vi "Open_File_Simple.vi"(6 "Read Only?":bool, 8 "error in (no error)":errorcluster, 9 "Overwrite?":bool, 10 "Path relative?":bool, 11 "Path":string) -> (0 "error out":errorcluster, 3 "refnum out":refnum<file>)   [LabVIEW 2016]
uses:
  <vilib>/Utility/error.llb/Error Cluster From Error Code.vi
  <vilib>/ErrorRing/Error Ring.xnode
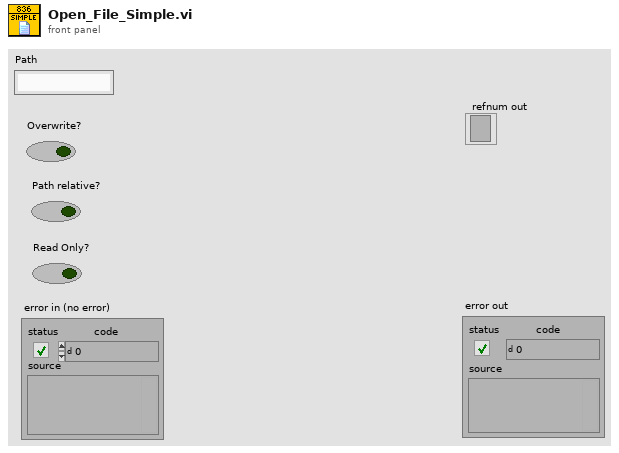
[diagram p1: front panel]
types:
  T1 = enum16{"open", "replace", "create", "open or create", "replace or create", "replace or create with confirmation"}
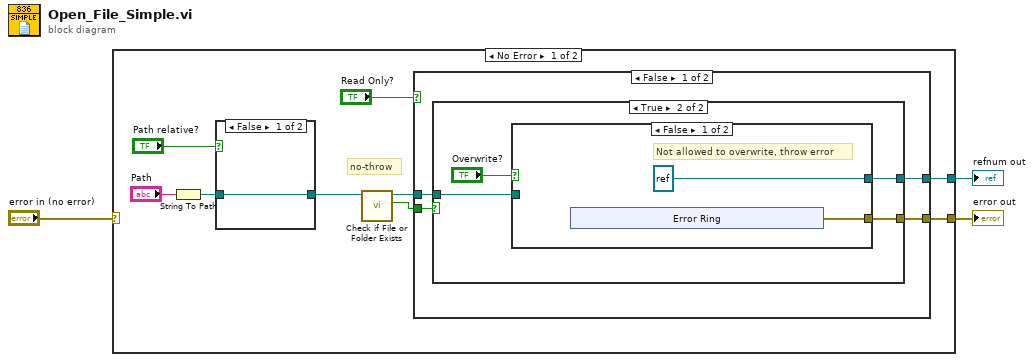
[diagram p0: block diagram]
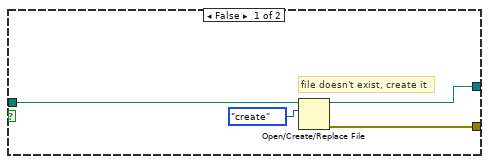
[diagram p2: hidden frame]
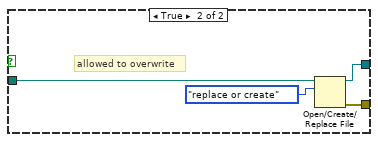
[diagram p3: hidden frame]
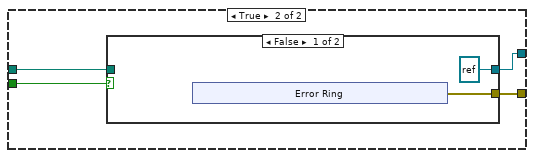
[diagram p4: hidden frame]
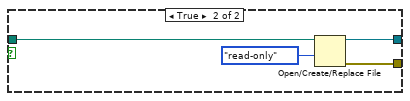
[diagram p5: hidden frame]
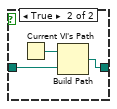
[diagram p6: hidden frame]
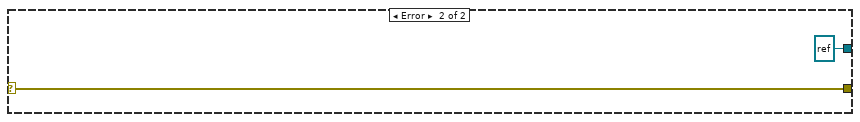
[diagram p7: hidden frame]
diagram:
  n1 = case shown="No Error" "error in (no error)" {
    selector: "error in (no error)" -> [_ w55]
    tunnel: [w5 w55] -> w2
    tunnel: [w4 refnum<file> refnum ("refnum out")] -> w1
    frame No Error {
      # "no-throw"
      n2 = String To Path(string="Path") -> (path=w11:path)
      n3 = case shown="False" "Path relative?" {
        tunnel: w11 -> [w50 w53]
        tunnel: [w50 w51] -> w12
        frame False {
        }
        frame True {
          n4 = Current VI's Path() -> (path=w52:path)
          n5 = Build Path(base path=w52, name or relative path=w53) -> (appended path=w51:path)
        }
      }
      n6 = call <vilib>:"Check if File or Folder Exists.vi"("path"=w12) -> ("file or folder exists?"=w7:bool, "dup path"=w8:path)  [unwired: 8 in, 1 out]
      n7 = case shown="False" "Read Only?" {
        tunnel: w8 -> [w16 w36]
        tunnel: w7 -> [w15 w39]
        tunnel: [w13 w38] -> w5
        tunnel: [w14 w37] -> w4
        frame False {
          n8 = case shown="True" w15 {
            tunnel: w16 -> [w20 w23]
            tunnel: [w18 w22] -> w13
            tunnel: [w19 w21] -> w14
            frame False {
              # "file doesn't exist, create it"
              n9 = Open/Create/Replace File(file path (use dialog)=w20, operation (0:open)=T1."create") -> (refnum out=w19:refnum<file>, error out=w18:errorcluster)  [unwired: 4 in, 1 out]
            }
            frame True {
              n10 = case shown="False" "Overwrite?" {
                tunnel: w23 -> [_ w34]
                tunnel: [w25 w32] -> w22
                tunnel: [refnum<file> refnum ("refnum out") w33] -> w21
                frame False {
                  # "Not allowed to overwrite, throw error"
                  n11 = xnode "Error Ring"() -> ("error out"=w25:errorcluster)
                }
                frame True {
                  # "allowed to overwrite"
                  n12 = Open/Create/Replace File(file path (use dialog)=w34, operation (0:open)=T1."replace or create") -> (refnum out=w33:refnum<file>, error out=w32:errorcluster)  [unwired: 4 in, 1 out]
                }
              }
            }
          }
        }
        frame True {
          n13 = case shown="False" w39 {
            tunnel: [w41 w46] -> w38
            tunnel: [refnum<file> refnum ("refnum out") w49] -> w37
            tunnel: w36 -> [_ w47]
            frame False {
              n14 = xnode "Error Ring"() -> ("error out"=w41:errorcluster)
            }
            frame True {
              n15 = Open/Create/Replace File(file path (use dialog)=w47, access (0:read/write)=enum16{"read/write", "read-only", "write-only"}."read-only") -> (refnum out=w49:refnum<file>, error out=w46:errorcluster)  [unwired: 4 in, 1 out]
            }
          }
        }
      }
    }
    frame Error {
    }
  }
  "error out" <- w2
  "refnum out" <- w1
